vi "DFConfig Write ROIS.vi"(8 "error in (no error)":errorcluster, 10 "Global Settings":T1={"Query Timeout (120)"=120, "Connection Timeout (30)"=30, "Indexer Idle Time (10)"=10, " Database Path (empty)"=path ""}, 11 "My.DataFinder In":string) -> (0 "error out":errorcluster, 1 "CrawlSettings ID":string, 2 "First CrawlDir ID":string, 3 "My.DataFinder Out":string)   [LabVIEW 2011]
uses:
  DFConfig GLOBAL.ctl
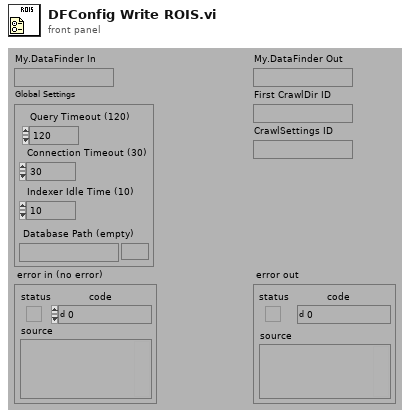
[diagram p1: front panel]
types:
  T1 = typedef "DFConfig GLOBAL.ctl" = cluster{"Query Timeout (120)":i32, "Connection Timeout (30)":i32, "Indexer Idle Time (10)":i32, " Database Path (empty)":path}
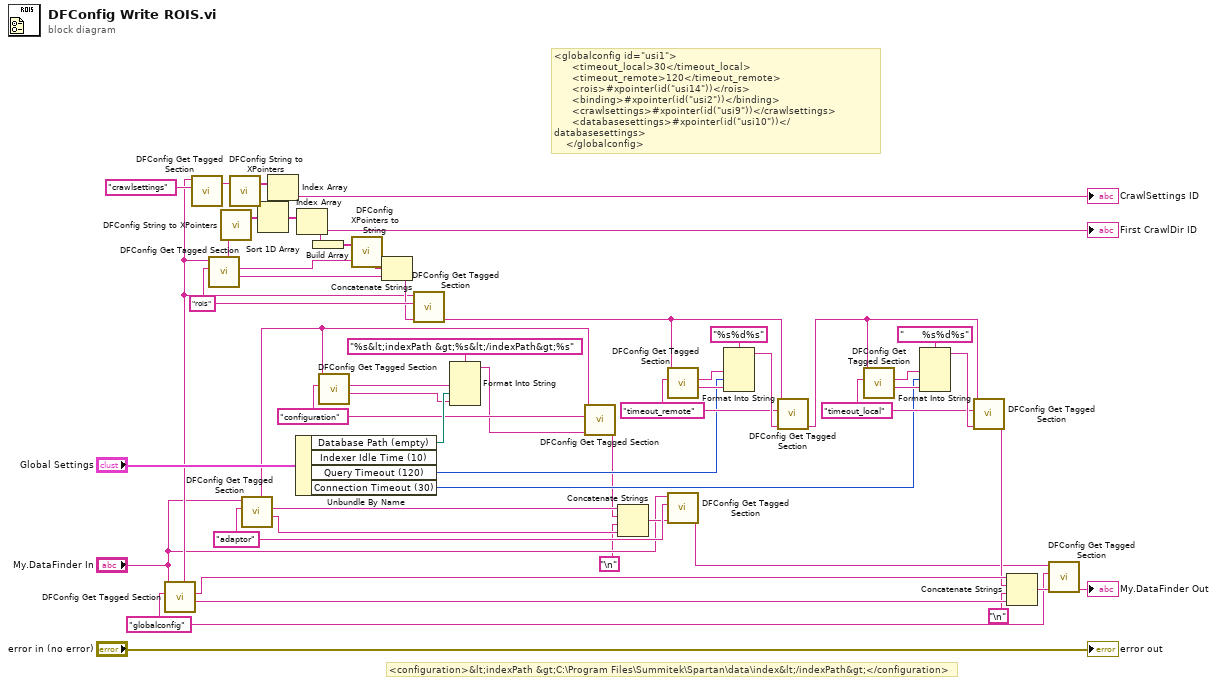
[diagram p0: block diagram]
diagram:
  w11 = "configuration" ("Tag (\"\")")
  w8 = "adaptor" ("Tag (\"\")")
  w25 = "timeout_remote" ("Tag (\"\")")
  w30 = "timeout_local" ("Tag (\"\")")
  w37 = "globalconfig" ("Tag (\"\")")
  w48 = "rois" ("Tag (\"\")")
  # "<configuration>&lt;indexPath &gt;C:\\Program Files\\Summitek\\Spartan\\data\\index&lt;/indexPath&gt;</configuration>"
  # "<globalconfig id=\"usi1\">\n      <timeout_local>30</timeout_local>\n      <timeout_remote>120</timeout_remote>\n      <rois>#xpointer(id(\"usi14\"))</rois>\n      <binding>#xpointer(id(\"usi2\"))</binding>\n      <crawlsettings>#xpointer(id(\"usi9\"))</crawlsettings>\n      <databasesettings>#xpointer(id(\"usi10\"))</databasesettings>\n    </globalconfig>"
  n1 = call "DFConfig Get Tagged Section.vi"("Tag (\"\")"=w37, "String"="My.DataFinder In") -> ("End Tag"=w39:string, "Start Tag"=w40:string, "InnerString"=w16:string)  [unwired: 1 in, 6 out]
  n2 = call "DFConfig Get Tagged Section.vi"("Tag (\"\")"="crawlsettings" ("Tag (\"\")"), "String"=w16) -> ("InnerString"=w42:string)  [unwired: 1 in, 8 out]
  n3 = call "DFConfig Get Tagged Section.vi"("Tag (\"\")"=w48, "String"=w16) -> ("End Tag"=w49:string, "Start Tag"=w51:string, "InnerString"=w52:string)  [unwired: 1 in, 6 out]
  n4 = call "DFConfig String to XPointers.vi"("String"=w52) -> ("Xpointers"=w34:string[])  [unwired: 2 out]
  n5 = call "DFConfig String to XPointers.vi"("String"=w42) -> ("Xpointers"=w43:string[])  [unwired: 2 out]
  n6 = call "DFConfig Get Tagged Section.vi"("Tag (\"\")"=w8, "String"="My.DataFinder In") -> ("End Tag"=w6:string, "Start Tag"=w7:string, "InnerString"=w9:string)  [unwired: 1 in, 6 out]
  n7 = Sort 1D Array(array=w34) -> (sorted array=w33:string[])
  n8 = Index Array(array=w43) -> (element=→"CrawlSettings ID":string)  [unwired: 1 in]
  n9 = Unbundle By Name("Global Settings") -> ("Database Path (empty)"=w14:path, "Query Timeout (120)"=w19:i32, "Connection Timeout (30)"=w21:i32)  [unwired: 1 out]
  n10 = Index Array(array=w33) -> (element=w45:string)  [unwired: 1 in]
  "First CrawlDir ID" <- w45
  n11 = Build Array(w45) -> (w46:string[])
  n12 = call "DFConfig Get Tagged Section.vi"("Tag (\"\")"=w11, "String"=w9) -> ("End Tag"=w12:string, "Start Tag"=w13:string)  [unwired: 1 in, 7 out]
  n13 = call "DFConfig XPointers to String.vi"("XPointers (empty)"=w46) -> ("xpointer"=w50:string)  [unwired: 2 out]
  n14 = Concatenate Strings(w51, w50, w49) -> (w47:string)
  n15 = call "DFConfig Get Tagged Section.vi"("Replacement String (\"\")"=w47, "Tag (\"\")"=w48, "String"=w16) -> ("String with Replacement"=w17:string)  [unwired: 8 out]
  n16 = Format Into String(format string="%s&lt;indexPath &gt;%s&lt;/indexPath&gt;%s" ("Tag (\"\")"), w13, w14, w12) -> (resulting string=w10:string)  [unwired: 2 in, 1 out]
  n17 = call "DFConfig Get Tagged Section.vi"("Replacement String (\"\")"=w10, "Tag (\"\")"=w11, "String"=w9) -> ("String with Replacement"=w5:string)  [unwired: 8 out]
  n18 = Concatenate Strings(w7, w5, "\n", w6) -> (w4:string)
  n19 = call "DFConfig Get Tagged Section.vi"("Tag (\"\")"=w25, "String"=w17) -> ("End Tag"=w22:string, "Start Tag"=w23:string)  [unwired: 1 in, 7 out]
  n20 = call "DFConfig Get Tagged Section.vi"("Replacement String (\"\")"=w4, "Tag (\"\")"=w8, "String"="My.DataFinder In") -> ("String with Replacement"=w2:string)  [unwired: 8 out]
  n21 = Format Into String(format string="%s%d%s" ("Tag (\"\")"), w23, w19, w22) -> (resulting string=w26:string)  [unwired: 2 in, 1 out]
  n22 = call "DFConfig Get Tagged Section.vi"("Replacement String (\"\")"=w26, "Tag (\"\")"=w25, "String"=w17) -> ("String with Replacement"=w18:string)  [unwired: 8 out]
  n23 = call "DFConfig Get Tagged Section.vi"("Tag (\"\")"=w30, "String"=w18) -> ("End Tag"=w27:string, "Start Tag"=w28:string)  [unwired: 1 in, 7 out]
  n24 = Format Into String(format string="      %s%d%s" ("Tag (\"\")"), w28, w21, w27) -> (resulting string=w31:string)  [unwired: 2 in, 1 out]
  n25 = call "DFConfig Get Tagged Section.vi"("Replacement String (\"\")"=w31, "Tag (\"\")"=w30, "String"=w18) -> ("String with Replacement"=w20:string)  [unwired: 8 out]
  n26 = Concatenate Strings(w40, w20, "\n", w39) -> (w38:string)
  n27 = call "DFConfig Get Tagged Section.vi"("Replacement String (\"\")"=w38, "Tag (\"\")"=w37, "String"=w2) -> ("String with Replacement"=→"My.DataFinder Out":string)  [unwired: 8 out]
  "error out" <- "error in (no error)"
